vi "RunJS3.vi"() -> ()   [LabVIEW 2013]
uses:
  System.Windows.Forms
  E:/Dropbox/ni/lvcef/github/lvcef/dotnet/LVCef/bin/Debug/LVCef.dll
  dotnet/LVCef/bin/Debug/LVCef.dll
  E:/Dropbox/ni/lvcef/github/lvcef/dotnet/LVCef/bin/Debug/Xilium.CefGlue.dll
  dotnet/LVCef/bin/Debug/Xilium.CefGlue.dll
panel:
  in  "ToolStripContainer":refnum<k24>(container)
  out "Numeric":i32
  in  "stop":bool
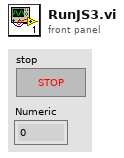
[diagram p1: front panel]
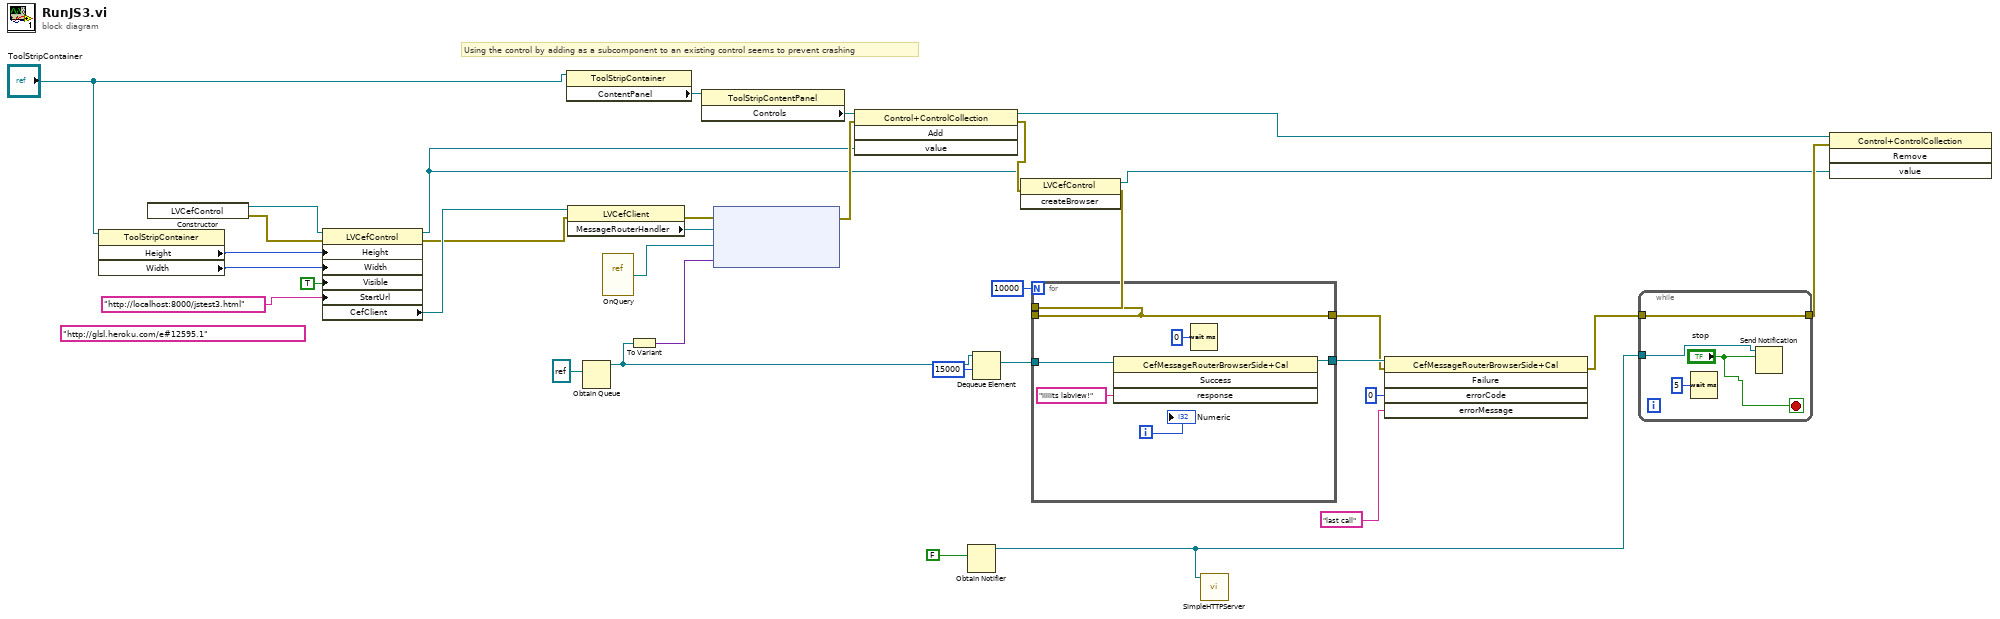
[diagram p0: block diagram]
diagram:
  (unwired) "http://glsl.heroku.com/e#12595.1" ("StartUrl")
  # "Using the control by adding as a subcomponent to an existing control seems to prevent crashing"
  n1 = property class="ToolStripContainer"(reference="ToolStripContainer") -> ("Height"=w23:i32, "Width"=w22:i32)  [unwired: 1 in, 2 out]
  n2 = constructor class="LVCefControl"() -> (reference out=w30:refnum<k24>, error out=w31:errorcluster)  [unwired: 3 in, 1 out]
  n3 = property class="LVCefControl"(reference=w30, error in=w31, "Height"=w23, "Width"=w22, "Visible"=TRUE, "StartUrl"="http://localhost:8000/jstest3.html") -> (reference out=w2:refnum<k24>, error out=w3:errorcluster, "CefClient"=w4:refnum<k24>)
  n4 = property class="ToolStripContainer"(reference="ToolStripContainer") -> ("ContentPanel"=w29:refnum<k24>)  [unwired: 1 in, 2 out]
  n5 = property class="LVCefClient"(reference=w4, error in=w3) -> (error out=w33:errorcluster, "MessageRouterHandler"=w32:refnum<k24>)  [unwired: 1 out]
  n6 = Obtain Queue(element data type=refnum<k24> refnum ("callback")) -> (queue out=w16:refnum<queue>)  [unwired: 4 in, 2 out]
  n7 = vi-ref "OnQuery.vi"() -> ("vi reference"=w20:refnum<vi>)
  n8 = To Variant(anything=w16) -> (Variant=w17:variant)
  n9 = property class="ToolStripContentPanel"(reference=w29) -> ("Controls"=w28:refnum<k24>)  [unwired: 1 in, 2 out]
  n10 = node(w33, w32, w20, w17) -> (w25:errorcluster)  [unwired: 1 in, 1 out]
  n11 = invoke class="Control+ControlCollection" method="Add"(reference=w28, error in=w25, "value"=w2) -> (reference out=w27:refnum<k24>, error out=w24:errorcluster)  [unwired: 1 in, 2 out]
  n12 = Obtain Notifier(notification data type=FALSE) -> (notifier out=w10:refnum<notifier>)  [unwired: 3 in, 2 out]
  n13 = Dequeue Element(queue=w16, timeout in ms (-1)=15000) -> (element=w15:refnum<k24>)  [unwired: 1 in, 3 out]
  n14 = invoke class="LVCefControl" method="createBrowser"(reference=w2, error in=w24) -> (reference out=w1:refnum<k24>, error out=w26:errorcluster)  [unwired: 1 in, 1 out]
  n15 = for {
    N: 10000 -> [_]
    tunnel: [w38] -> _
    tunnel: [w38] -> w6
    tunnel: w26 -> [w38]
    tunnel: w15 -> [w37]
    tunnel: [w35] -> w9
    i -> [w40]
    n16 = invoke class="CefMessageRouterBrowserSide+Cal" method="Success"(reference=w37, "response"="iiiiits labview!") -> (reference out=w35:refnum<k24>)  [unwired: 2 in, 3 out]
    n17 = Wait (ms)(milliseconds to wait=u32 0) -> ()  [unwired: 1 out]
    "Numeric" <- w40
  }
  n18 = call "SimpleHTTPServer.vi"("Stop Notifier"=w10) -> ()  [unwired: 10 in, 1 out]
  n19 = invoke class="CefMessageRouterBrowserSide+Cal" method="Failure"(reference=w9, error in=w6, "errorCode"=0, "errorMessage"="last call") -> (error out=w5:errorcluster)  [unwired: 1 in, 4 out]
  n20 = while {
    tunnel: w5 -> [w44]
    tunnel: [w44] -> w11
    tunnel: w10 -> [w43]
    stop <- "stop" stop-if-true
    n21 = Wait (ms)(milliseconds to wait=u32 5) -> ()  [unwired: 1 out]
    n22 = Send Notification(notification="stop", notifier=w43) -> ()  [unwired: 1 in, 2 out]
  }
  n23 = invoke class="Control+ControlCollection" method="Remove"(reference=w27, error in=w11, "value"=w1) -> ()  [unwired: 1 in, 4 out]
